vi "Get other terminals on wire.vi"(8 "error in (no error)":errorcluster, 11 "Reference":refnum<vi>) -> (0 "error out":errorcluster, 1 "Wire":refnum<vi>, 2 "Sink Terminals":refnum<vi>[](array[refnum]), 3 "Source Terminal":refnum<vi>)   [LabVIEW 2012, in "Scripting Tools.lvlib"]
doc: "Get the wire connected to the first terminal of <b>Reference</b> and find all the terminals connected to this wire - one <b>Source Terminal</b> and multiple <b>Sink Terminals</b>"
uses:
  <userlib>/_LAVAcr/Scripting Tools/Scripting Tools.lvlib
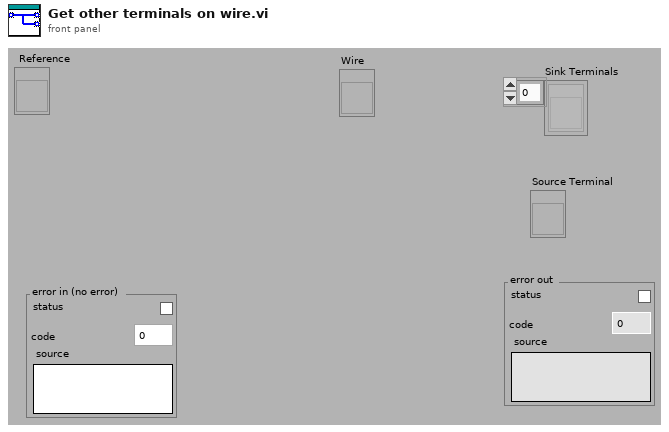
[diagram p1: front panel]
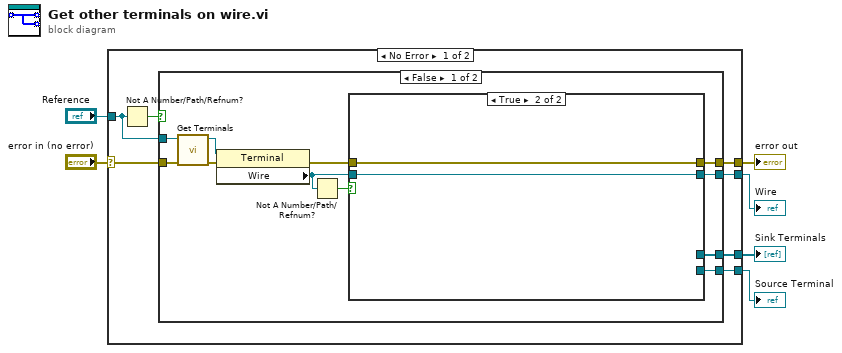
[diagram p0: block diagram]
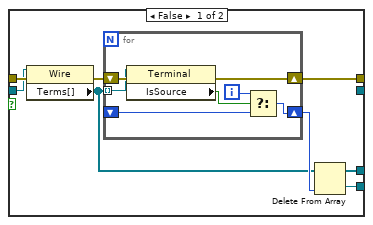
[diagram p2: hidden frame]
diagram:
  n1 = case shown="No Error" "error in (no error)" {
    selector: "error in (no error)" -> [w10 w43]
    tunnel: [w13 _] -> w5
    tunnel: [w12 _] -> w4
    tunnel: [w11 w43] -> w3
    tunnel: "Reference" -> [w9 _]
    tunnel: [w7 _] -> w1
    frame No Error {
      n2 = Not A Number/Path/Refnum?(number/path/refnum=w9) -> (NaN/Path/Refnum?=w8:bool)
      n3 = case shown="False" w8 {
        tunnel: [w23 _] -> w13
        tunnel: [w22 _] -> w12
        tunnel: [w21 w42] -> w11
        tunnel: w10 -> [w18 w42]
        tunnel: w9 -> [w17 _]
        tunnel: [w14 _] -> w7
        frame False {
          n4 = call "Get Terminals.vi"("error in (no error)"=w18, "Reference"=w17) -> ("error out"=w20:errorcluster, "First Terminal"=w19:refnum<vi>)  [unwired: 8 out]
          n5 = property class="Terminal"(reference=w19, error in=w20) -> (error out=w24:errorcluster, "Wire"=w15:refnum<vi>)  [unwired: 1 out]
          n6 = Not A Number/Path/Refnum?(number/path/refnum=w15) -> (NaN/Path/Refnum?=w16:bool)
          n7 = case shown="True" w16 {
            tunnel: w24 -> [w32 w41]
            tunnel: w15 -> [w31 w40]
            tunnel: [w27 _] -> w23
            tunnel: [w26 _] -> w22
            tunnel: [w25 w41] -> w21
            tunnel: [_ w40] -> w14
            frame False {
              n8 = property class="Wire"(reference=w31, error in=w32) -> (error out=w30:errorcluster, "Terms[]"=w28:refnum<vi>[])  [unwired: 1 out]
              n9 = for {
                shift-right: [w33] -> w25
                shift-left: w30 -> [w39]
                tunnel: w28 -> [w38] mode=indexing
                shift-right: [w35] -> w29
                shift-left: _ -> [w34]
                i -> [w36]
                n10 = property class="Terminal"(reference=w38, error in=w39) -> (error out=w33:errorcluster, "IsSource"=w37:bool)  [unwired: 1 out]
                n11 = Select(t=w36, s=w37, f=w34) -> (s? t:f=w35:i32)
              }
              n12 = Delete From Array(array=w28, index=w29) -> (deleted portion=w26:refnum<vi>, array with subset deleted=w27:refnum<vi>[])  [unwired: 1 in]
            }
            frame True {
            }
          }
        }
        frame True {
        }
      }
    }
    frame Error {
    }
  }
  "error out" <- w3
  "Sink Terminals" <- w5
  "Source Terminal" <- w4
  "Wire" <- w1
